vi "Logger.Add.vi"(8 "error in":errorcluster, 10 "HandledFileContent":T1 {"Values" format="%.3f"}, 11 "Refnum in":refnum<k34>) -> (0 "error out":errorcluster, 3 "Refnum out":refnum<k34>)   [LabVIEW 2016]
uses:
  Logger.FileBody.ctl
  Global/ApplicationGlobal.vi
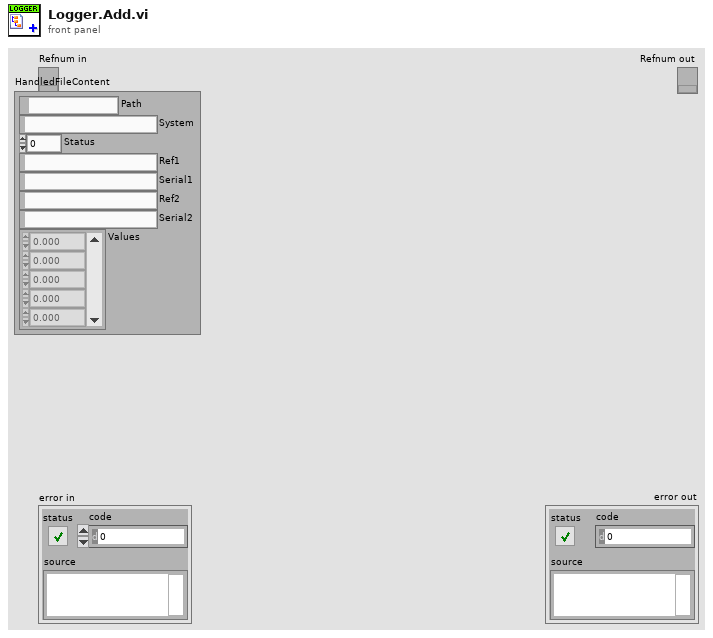
[diagram p1: front panel]
types:
  T1 = typedef "Logger.FileBody.ctl" = cluster{"Path":path, "System":string, "Status":u8, "Ref1":string, "Serial1":string, "Ref2":string, "Serial2":string, "Values":sgl[]}
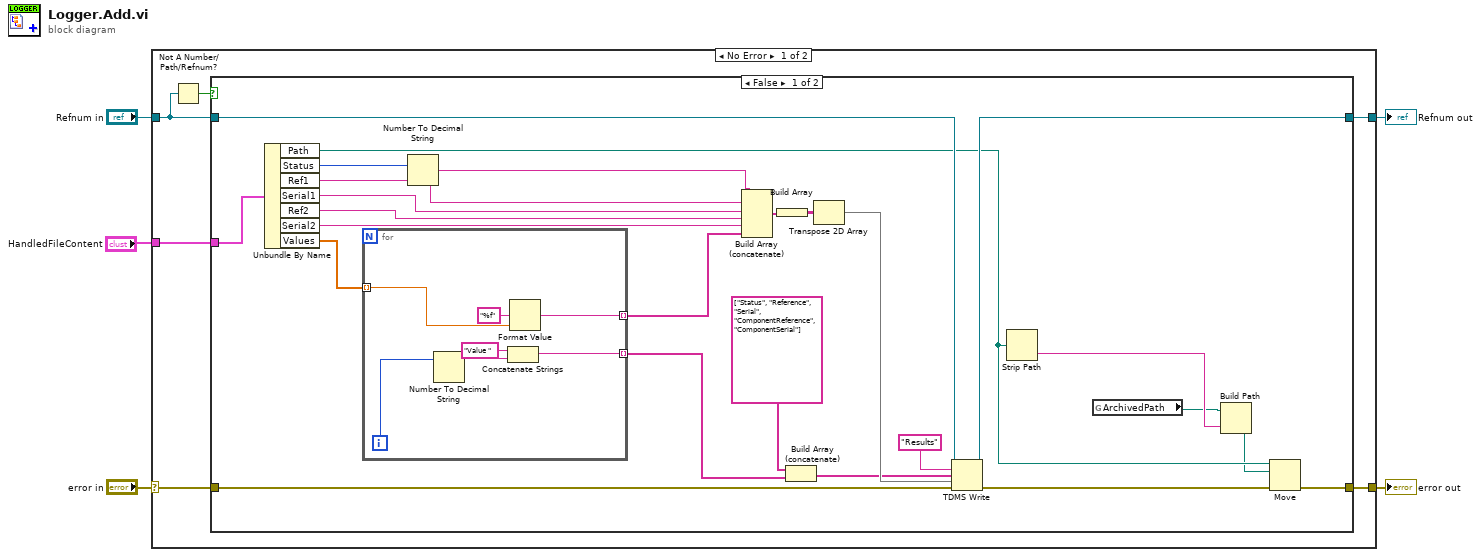
[diagram p0: block diagram]
diagram:
  n1 = case shown="No Error" "error in" {
    selector: "error in" -> [w11 w47]
    tunnel: [w9 w46] -> w5
    tunnel: [w10 w47] -> w4
    tunnel: "Refnum in" -> [w8 w46]
    tunnel: "HandledFileContent" -> [w6 _]
    frame No Error {
      n2 = Not A Number/Path/Refnum?(number/path/refnum=w8) -> (NaN/Path/Refnum?=w7:bool)
      n3 = case shown="False" w7 {
        tunnel: w11 -> [w34 w44]
        tunnel: [w15 w44] -> w10
        tunnel: [w35 w45] -> w9
        tunnel: w8 -> [w36 w45]
        tunnel: w6 -> [w31 _]
        frame False {
          n4 = Unbundle By Name(w31) -> ("Path"=w16:path, "Status"=w30:u8, "Ref1"=w28:string, "Serial1"=w27:string, "Ref2"=w26:string, "Serial2"=w25:string, "Values"=w24:sgl[])
          n5 = for {
            tunnel: w24 -> [w40] mode=indexing
            tunnel: [w38] -> w23 mode=indexing
            tunnel: [w37] -> w21 mode=indexing
            i -> [w43]
            n6 = Number To Decimal String(number=w43) -> (decimal integer string=w42:string)  [unwired: 1 in]
            n7 = Concatenate Strings("Value " ("string"), w42) -> (w37:string)
            n8 = Format Value(format string="%f", value (0)=w40) -> (output string=w38:string)  [unwired: 1 in]
          }
          n9 = Number To Decimal String(number=w30) -> (decimal integer string=w29:string)  [unwired: 1 in]
          n10 = Build Array (concatenate)(w29, w28, w27, w26, w25, w23) -> (w19:string[])
          n11 = Build Array(w19) -> (w18:string[][])
          n12 = Build Array (concatenate)(string[] ["Status", "Reference", "Serial", "ComponentReference", "ComponentSerial"] ("channel name(s) in (Untitled)"), w21) -> (w20:string[])
          n13 = Transpose 2D Array(2D array=w18) -> (transposed array=w32:string[][])
          n14 = TDMS Write(0:w36, 5:"Results" ("group name in (Untitled)"), 7:w20, 9:w32, 11:w34) -> (4:w35:refnum<k34>, 15:w17:errorcluster)  [unwired: 1 in, 2 out]
          n15 = Strip Path(path=w16) -> (name=w13:string)  [unwired: 1 out]
          n16 = global read "ApplicationGlobal.vi" "ArchivedPath"() -> (w12:path)
          n17 = Build Path(base path=w12, name or relative path=w13) -> (appended path=w14:path)
          n18 = Move(source path=w16, error in=w17, 10:w14) -> (error out=w15:errorcluster)  [unwired: 2 in, 2 out]
        }
        frame True {
        }
      }
    }
    frame Error {
    }
  }
  "Refnum out" <- w5
  "error out" <- w4
